vi "CreatePublicEvents.vi"(8 "error in (no error)":errorcluster, 11 "SMO.Dictionary":refnum<class "SMO.Dictionary.lvclass">) -> (0 "error out":errorcluster, 3 "SMO.Dictionary out":refnum<class "SMO.Dictionary.lvclass">)   [LabVIEW 2013, in "SMO.Dictionary.lvlib" / "SMO.Dictionary.lvclass"]
doc: "JKI State Machine Objects (SMO) 1.0.1.12\nJKI - JKI\nCopyright (c) 2016, JKI"
uses:
  SMO.Dictionary.lvclass
  Typedefs/PrivateEvents--SMO.Dictionary.KeyValue-Pair.ctl
  SMO.Dictionary.lvclass/SMO.Dictionary.ctl
  <vilib>/JKI/JKI SMO/SMO/SMO.lvclass
panel:
  # "For instructions on how to use the JKI State Machine Objects, examples and video tutorials, visit:\nhttp://jki.net/state-machine-objects/\n\nJKI State Machine Objects™\nhttp://jki.net/state-machine-objects/\nCopyright (C) 2005-2015, JKI <info@jki.net>\nALL RIGHTS RESERVED"
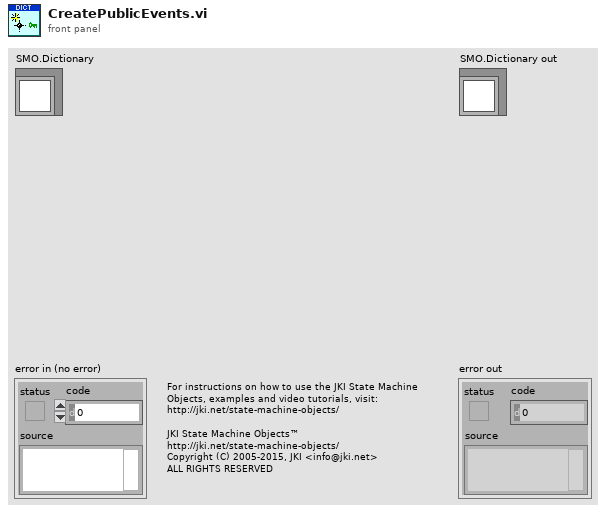
[diagram p1: front panel]
types:
  T1 = typedef "SMO.Dictionary.lvlib/SMO.Dictionary.lvclass/PrivateEvents--SMO.Dictionary.KeyValue-Pair.ctl" = cluster{"Key":string, "Value":variant}
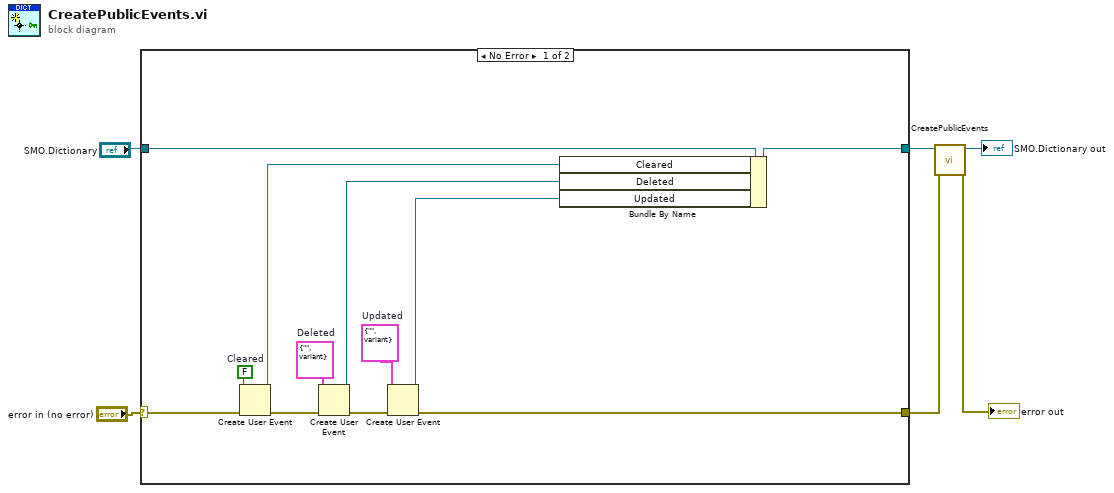
[diagram p0: block diagram]
diagram:
  n1 = case shown="No Error" "error in (no error)" {
    selector: "error in (no error)" -> [w17 w20]
    tunnel: [w8 w20] -> w2
    tunnel: [w16 w19] -> w3
    tunnel: "SMO.Dictionary" -> [w18 w19]
    frame No Error {
      w10 = T1 {"Key"="", "Value"=variant}  # Updated
      w13 = FALSE  # Cleared
      w15 = T1 {"Key"="", "Value"=variant}  # Deleted
      n2 = Create User Event(user event datatype=w13, error in=w17) -> (user event=w12:refnum<user-event>, error out=w14:errorcluster)
      n3 = Create User Event(user event datatype=w15, error in=w14) -> (user event=w11:refnum<user-event>, error out=w9:errorcluster)
      n4 = Create User Event(user event datatype=w10, error in=w9) -> (user event=w7:refnum<user-event>, error out=w8:errorcluster)
      n5 = Bundle By Name(cluster=w18, "Cleared"=w12, "Deleted"=w11, "Updated"=w7) -> (w16:refnum<class "SMO.Dictionary.lvclass">)
    }
    frame Error {
    }
  }
  n6 = call-parent "CreatePublicEvents.vi"("error in (no error)"=w2, "SMO"=w3) -> ("error out"=→"error out":errorcluster, "SMO out"=→"SMO.Dictionary out":refnum<class "SMO.Dictionary.lvclass">)  [unwired: 8 in]
